vi "Get Intermediate Result.vi"(8 "error in (no error)":errorcluster, 11 "AbstractCollector in":refnum<class "AbstractCollector.lvclass">) -> (0 "error out":errorcluster, 2 "AbstractData.lvclass":refnum<class "AbstractData.lvclass">, 3 "AbstractCollector out":refnum<class "AbstractCollector.lvclass">)   [LabVIEW 2014, in "AbstractCollector.lvclass"]
uses:
  AbstractCollector.lvclass
  Model/Data/AbstractData/AbstractData.lvclass
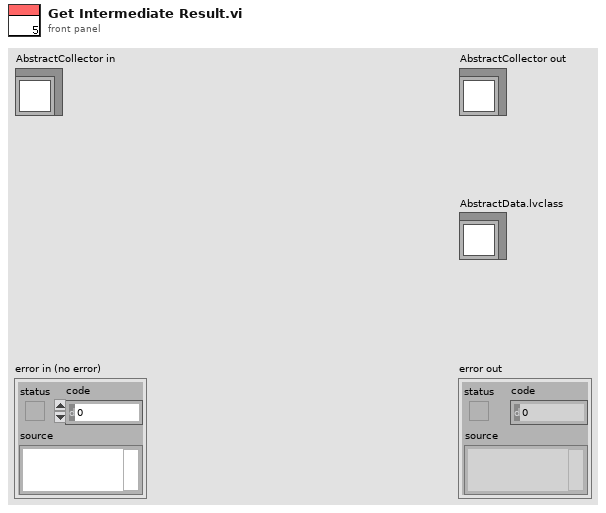
[diagram p1: front panel]
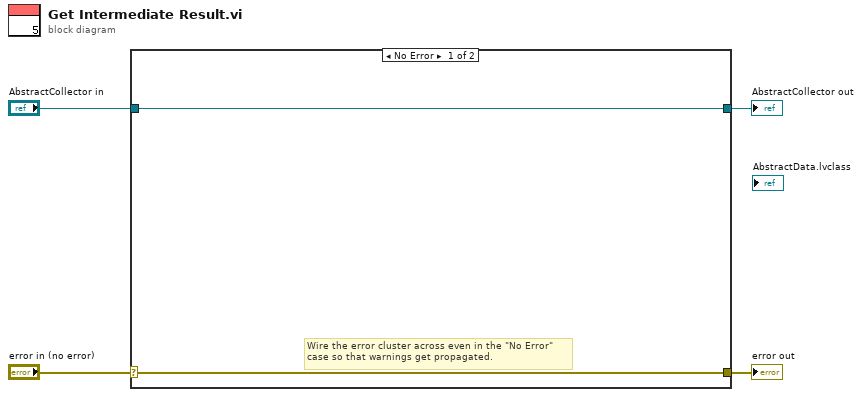
[diagram p0: block diagram]
diagram:
  n1 = case shown="No Error" "error in (no error)" {
    selector: "error in (no error)" -> [w5 w8]
    tunnel: [w5 w8] -> w3
    tunnel: [w6 w7] -> w1
    tunnel: "AbstractCollector in" -> [w6 w7]
    frame No Error {
      # "Wire the error cluster across even in the \"No Error\"\ncase so that warnings get propagated."
    }
    frame Error {
    }
  }
  "error out" <- w3
  "AbstractCollector out" <- w1
